vi "Kelvinox_Queue_Commands.vi"(1 "Control":T1, 3 "Queue":refnum<queue>) -> (0 "New Status":T1)   [LabVIEW 2019]
uses:
  Kelvinox/Kelvinox_Control.ctl
panel:
  # "Pressures in mbar"
  # "Temperatures in K"
  # "Pressures in mbar"
  # "Temperatures in K"
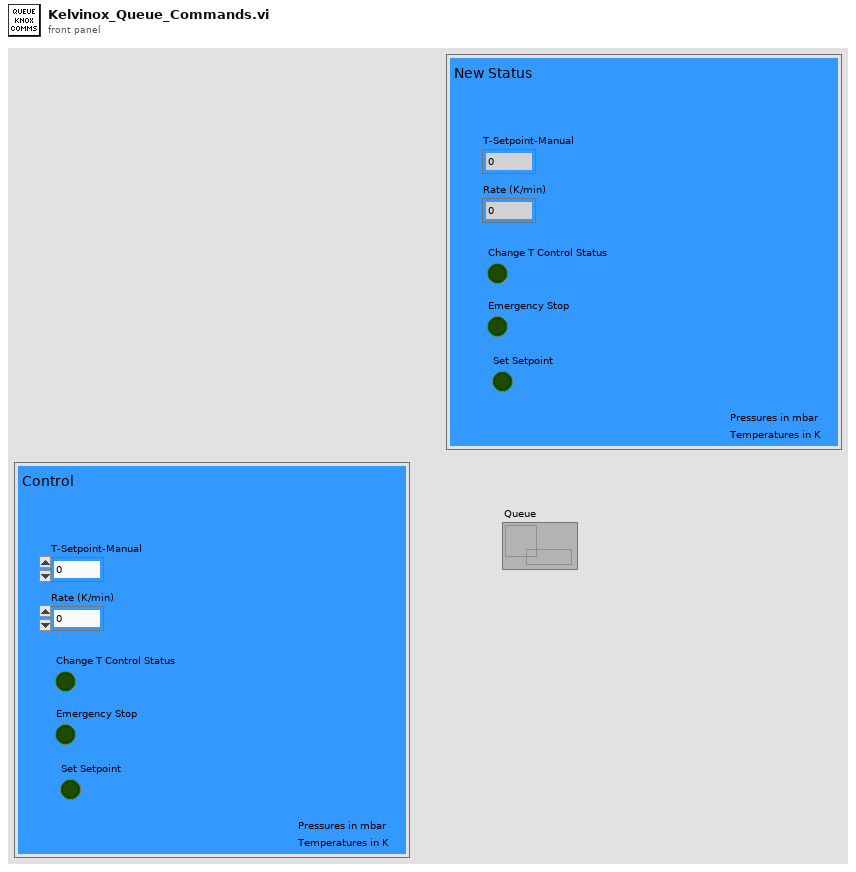
[diagram p1: front panel]
types:
  T1 = typedef "Kelvinox_Control.ctl" = cluster{"T-Setpoint-Manual":dbl, "Rate (K/min)":dbl, "Change T Control Status":bool, "Emergency Stop":bool, "Set Setpoint":bool}
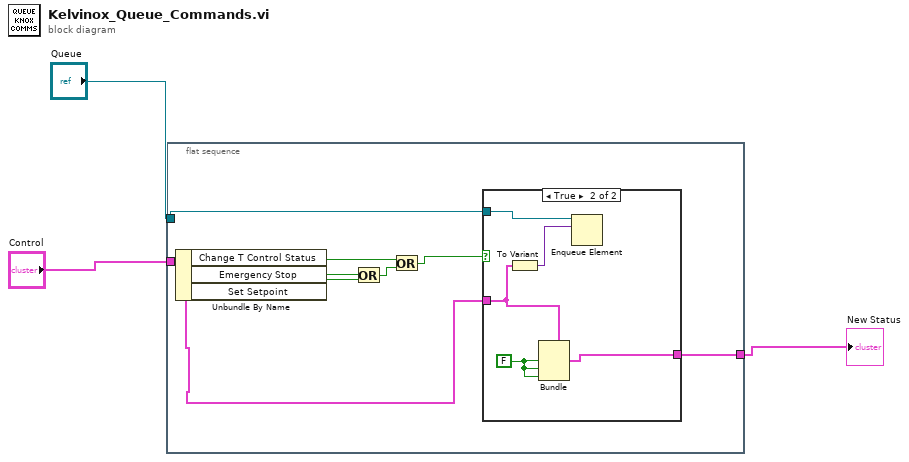
[diagram p0: block diagram]
diagram:
  n1 = flat-sequence {
    tunnel: "Queue" -> [w11]
    tunnel: "Control" -> [w7]
    tunnel: [w10] -> w2
    frame #0 {
      n2 = Unbundle By Name(w7) -> ("Change T Control Status"=w9:bool, "Emergency Stop"=w6:bool, "Set Setpoint"=w5:bool)
      n3 = Or(x=w6, y=w5) -> (x .or. y?=w4:bool)
      n4 = Or(x=w9, y=w4) -> (x .or. y?=w8:bool)
      n5 = case shown="True" w8 {
        tunnel: w11 -> [_ w17]
        tunnel: w7 -> [w12 w15]
        tunnel: [w12 w14] -> w10
        frame False {
        }
        frame True {
          w13 = FALSE
          n6 = To Variant(anything=w15) -> (Variant=w16:variant)
          n7 = Bundle(cluster=w15, "Change T Control Status"=w13, "Emergency Stop"=w13, "Set Setpoint"=w13) -> (w14:T1)  [unwired: 2 in]
          n8 = Enqueue Element(queue=w17, element=w16) -> ()  [unwired: 2 in, 3 out]
        }
      }
    }
  }
  "New Status" <- w2
